vi "find_path.vi"() -> ()   [LabVIEW 2019]
uses:
  karte/Koordinate.ctl
  karte/Karte.ctl
  karte/Kreuzung.ctl
  karte/Strasse.ctl
  karte/Verbindung.ctl
  karte/Strassentyp.ctl
  karte/Haus.ctl
  point_mode.ctl
  <vilib>/robotics/Navigation/shared/MapNode/DirectedGraphMapNode/NI_Robotics_DirectedGraphMapNode.lvclass
  C:/Program Files (x86)/National Instruments/LabVIEW 2019/vi.lib/robotics/Navigation/shared/MapNode/AbstractDstarNode/NI_Robotics_AbstractDstarNode.lvclass
  <vilib>/robotics/Navigation/shared/WorldMap/DirectedGraphWorldMap/NI_Robotics_DirectedGraphWorldMap.lvclass
  C:/Program Files (x86)/National Instruments/LabVIEW 2019/vi.lib/robotics/Navigation/shared/WorldMap/AbstractDstarWorldMap/NI_Robotics_AbstractDstarWorldMap.lvclass
  <vilib>/robotics/Navigation/shared/MapNode/AbstractDstarNode/NI_Robotics_AbstractDstarNode.lvclass
  C:/Program Files (x86)/National Instruments/LabVIEW 2019/vi.lib/robotics/Navigation/shared/MapNode/AbstractAstarNode/NI_Robotics_AbstractAstarNode.lvclass
  <vilib>/Utility/xml.llb/Read From XML File(array).vi
  <vilib>/robotics/Navigation/Anytime D Star/NI_Robotics_AnytimeDStar.lvclass
panel:
  out "error out":errorcluster
  out "nodes":cluster{"name":string, "coordinates":dbl[]}[](array[cluster])
  in  "Ziel Koord":T1={"x"=240.0, "y"=320.0}
  in  "Start Koord":T1={"x"=180.0, "y"=210.0}
  in  "file (use dialog)":path=path "\\\\fsamu18.adm.ds.fhnw.ch\\a_18_home12$/juerg.keller1/STUDPROJ/2019_2020/APAS/labview/karte/Parcelcity_Training_V2.3.xml"
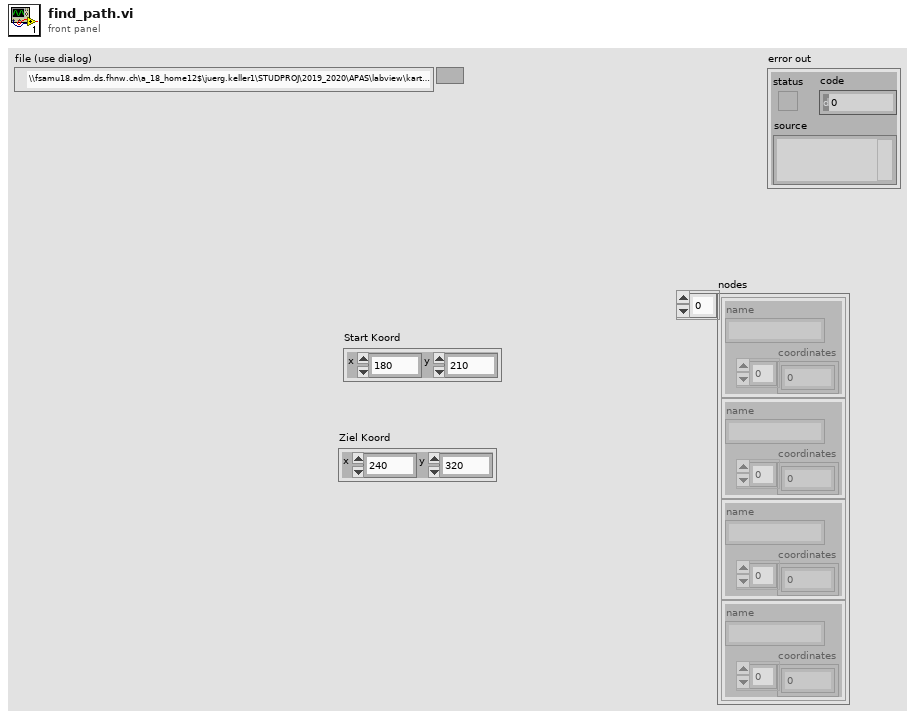
[diagram p1: front panel]
types:
  T1 = typedef "Koordinate.ctl" = cluster{"x":dbl, "y":dbl}
  T2 = typedef "point_mode.ctl" = enum16{"start", "end", "both"}
  T3 = typedef "Karte.ctl" = cluster{"Kreuzungen":T4[], "Strassen":T5[], "Häuser":T8[]}
  T4 = typedef "Kreuzung.ctl" = cluster{"Name":string, "Identifikation":u8, "Koord":T1, "Anzahl Abgänge":u8}
  T5 = typedef "Strasse.ctl" = cluster{"Name":string, "Identifikation":u8, "Verbindungen":T6[], "Breite":u8, "Strassen_Typ":T7}
  T6 = typedef "Verbindung.ctl" = cluster{"Start_Kr":u16, "Ziel_Kr":u16}
  T7 = typedef "Strassentyp.ctl" = enum16{"Innenstadt", "Stadt", "Land"}
  T8 = typedef "Haus.ctl" = cluster{"Name":string, "Hausnummer":u8, "Polygon":T1[], "Strassennummer":u8, "Türe":T1}
  T9 = typedef "2_Pt_Strasse.ctl" = cluster{"P1":T1, "P2":T1, "horizontal":bool}
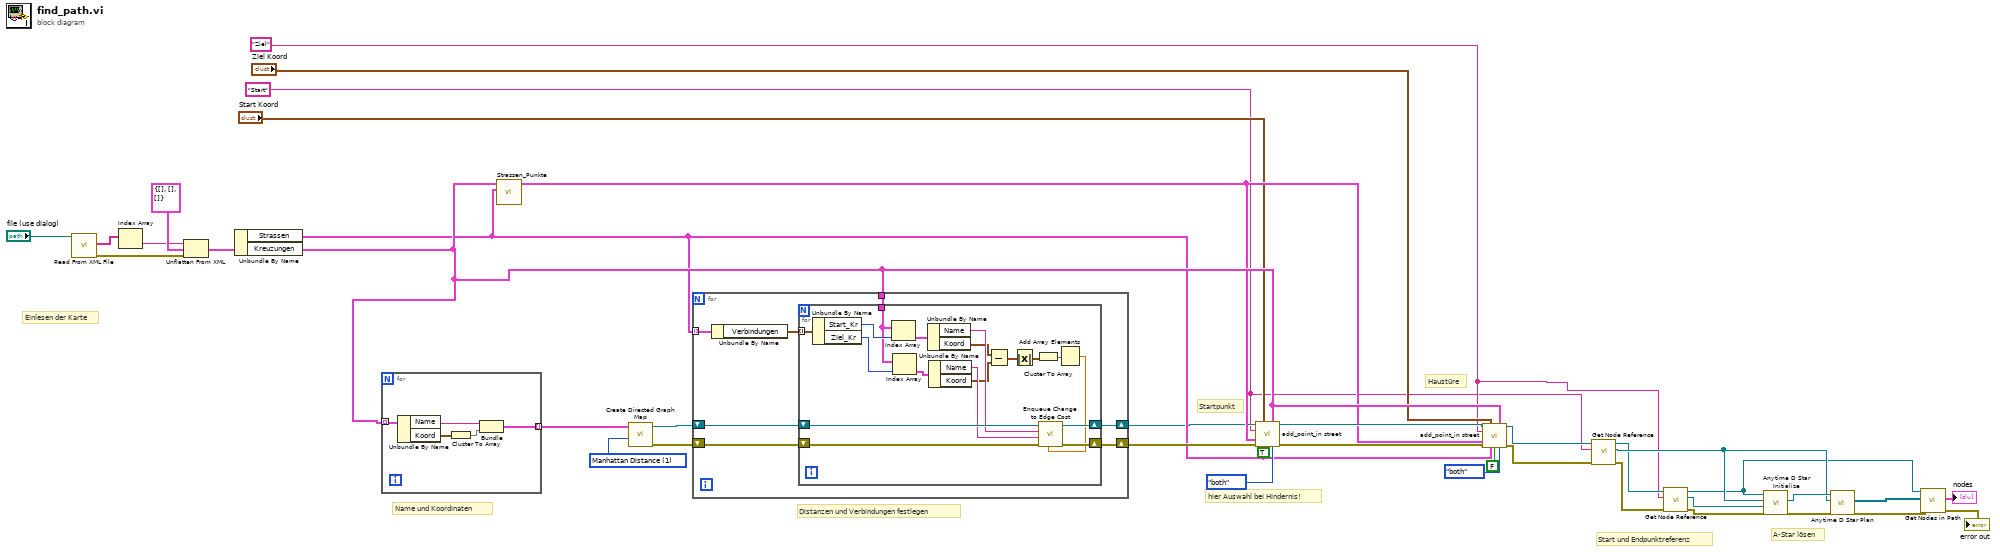
[diagram p0: block diagram]
diagram:
  w4 = "Ziel" ("name")
  w3 = "Start" ("name")
  w33 = u16 1 items=["Euclidean Distance", "Manhattan Distance"] ("heuristic function")
  # "A-Star lösen"
  # "Start und Endpunktreferenz"
  # "Haustüre"
  # "Startpunkt"
  # "Distanzen und Verbindungen festlegen"
  # "Name und Koordinaten"
  # "Einlesen der Karte"
  # "hier Auswahl bei Hindernis!"
  n1 = call-poly <vilib>:"Read From XML File.vi"("XML File Path"="file (use dialog)") -> ("error out"=w37:errorcluster, "XML Elements"=w38:string[])  [unwired: 8 in, 1 out]
  n2 = Index Array(array=w38) -> (element=w24:string)  [unwired: 1 in]
  n3 = Unflatten From XML(xml string=w24, type=T3 {"Kreuzungen"=[], "Strassen"=[], "Häuser"=[]} ("Karte"), error in (no error)=w37) -> (value=w35:T3)  [unwired: 1 out]
  n4 = Unbundle By Name(w35) -> ("Strassen"=w11:T5[], "Kreuzungen"=w12:T4[])
  n5 = for {
    tunnel: w12 -> [w44] mode=indexing
    tunnel: [w41] -> w34 mode=indexing
    n6 = Unbundle By Name(w44) -> ("Name"=w40:string, "Koord"=w43:T1)
    n7 = Cluster To Array(cluster=w43) -> (array=w42:dbl[])
    n8 = Bundle("Name"=w40, "Koord"=w42) -> (w41:cluster{"Name":string, "Koord":dbl[]})  [unwired: 1 in]
  }
  n9 = call "Strassen_Punkte.vi"("Strassen"=w11, "Kreuzungen"=w12) -> ("Strassenpunkte"=w10:T9[])  [unwired: 9 in]
  n10 = call <vilib>:"Create Directed Graph Map.vi"("heuristic function"=w33, "nodes"=w34) -> ("error out"=w18:errorcluster, "map reference out"=w19:refnum<data-value>)  [unwired: 8 in]
  n11 = for {
    shift-right: [w49] -> w7
    shift-left: w19 -> [w51]
    shift-right: [w48] -> w17
    shift-left: w18 -> [w50]
    tunnel: w11 -> [w47] mode=indexing
    tunnel: w12 -> [w45]
    n12 = Unbundle By Name(w47) -> ("Verbindungen"=w46:T6[])
    n13 = for {
      shift-right: [w67] -> w49
      shift-left: w51 -> [w69]
      shift-right: [w66] -> w48
      shift-left: w50 -> [w68]
      tunnel: w46 -> [w65] mode=indexing
      tunnel: w45 -> [w63]
      n14 = Unbundle By Name(w65) -> ("Start_Kr"=w64:u16, "Ziel_Kr"=w62:u16)
      n15 = Index Array(array=w63, index=w64) -> (element=w61:T4)
      n16 = Index Array(array=w63, index=w62) -> (element=w60:T4)
      n17 = Unbundle By Name(w61) -> ("Name"=w59:string, "Koord"=w56:T1)
      n18 = Unbundle By Name(w60) -> ("Name"=w58:string, "Koord"=w57:T1)
      n19 = Subtract(x=w56, y=w57) -> (x-y=w55:T1)
      n20 = Absolute Value(x=w55) -> (abs(x)=w54:T1)
      n21 = Cluster To Array(cluster=w54) -> (array=w53:dbl[])
      n22 = Add Array Elements(numeric array=w53) -> (sum=w52:dbl)
      n23 = call <vilib>:"Enqueue Change to Edge Cost.vi"("cost"=w52, "error in (no error)"=w68, "end node"=w58, "start node"=w59, "map reference in"=w69) -> ("error out"=w66:errorcluster, "map reference out"=w67:refnum<data-value>)  [unwired: 4 in]
    }
  }
  n24 = call "add_point_in street.vi"("Data Value Reference in"=w7, "Start Koord"="Start Koord", "Kreuzungen"=w12, "name"=w3, "Strassenpunkte"=w10, "error in (no error)"=w17, "Strassen"=w11, "Start"=TRUE, "mode"=point_mode."both") -> ("Data Value Reference out"=w15:refnum<data-value>, "error out"=w14:errorcluster)  [unwired: 5 in]
  n25 = call "add_point_in street.vi"("Data Value Reference in"=w15, "Start Koord"="Ziel Koord", "Kreuzungen"=w12, "name"=w4, "Strassenpunkte"=w10, "error in (no error)"=w14, "Strassen"=w11, "Start"=FALSE, "mode"=point_mode."both") -> ("Data Value Reference out"=w8:refnum<data-value>, "error out"=w13:errorcluster)  [unwired: 5 in]
  n26 = call <vilib>:"Get Node Reference.vi"("error in (no error)"=w13, "name"=w3, "map reference in"=w8) -> ("error out"=w32:errorcluster, "node reference"=w27:refnum<data-value>, "map reference out"=w21:refnum<data-value>)  [unwired: 5 in, 1 out]
  n27 = call <vilib>:"Get Node Reference.vi"("error in (no error)"=w32, "name"=w4, "map reference in"=w21) -> ("error out"=w30:errorcluster, "node reference"=w31:refnum<data-value>, "map reference out"=w20:refnum<data-value>)  [unwired: 5 in, 1 out]
  n28 = call <vilib>:"Anytime D Star Initialize.vi"("error in (no error)"=w30, "goal reference"=w31, "start reference"=w27, "map reference in"=w20) -> ("error out"=w28:errorcluster, "Anytime D*"=w29:refnum<class "NI_Robotics_AnytimeDStar.lvclass">)  [unwired: 6 in]
  n29 = call <vilib>:"Anytime D Star Plan.vi"("error in (no error)"=w28, "current reference"=w27, "Anytime D* in"=w29) -> ("error out"=w23:errorcluster, "path references"=w26:refnum<data-value>[])  [unwired: 4 in, 3 out]
  n30 = call <vilib>:"Get Nodes in Path.vi"("error in (no error)"=w23, "path references"=w26, "map reference in"=w20) -> ("error out"=→"error out":errorcluster, "nodes"=→"nodes":cluster{"name":string, "coordinates":dbl[]}[])  [unwired: 6 in, 1 out]
